vi "直通基准_数据库操作.vi"(8 "出口":i32, 9 "进口":i32, 11 "Freq&S":T1) -> ()   [LabVIEW 2015]
uses:
  network_Global/Global.vi
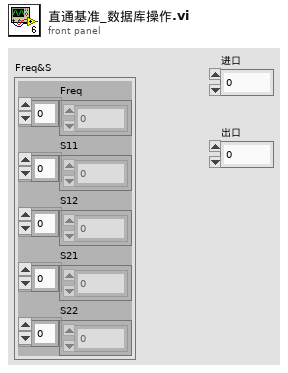
[diagram p1: front panel]
types:
  T1 = cluster{"Freq":dbl[], "S11":dbl[], "S12":dbl[], "S21":dbl[], "S22":dbl[]}
  T2 = typedef "测试类型.ctl" = u16
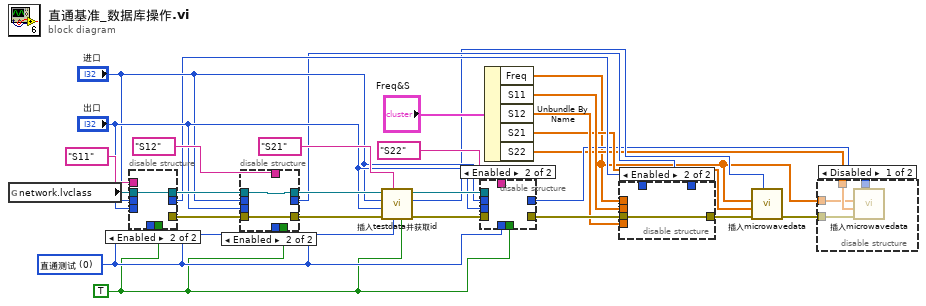
[diagram p0: block diagram]
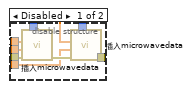
[diagram p3: hidden frame]
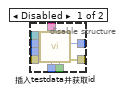
[diagram p4: hidden frame]
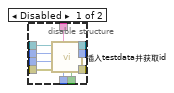
[diagram p5: hidden frame]
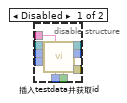
[diagram p6: hidden frame]
diagram:
  w2 = T2 0 items=["直通测试", "校准测试", "电缆"] ("测试类型")
  w1 = TRUE ("Ref")
  n1 = global read "Global.vi" "network.lvclass"() -> (w28:refnum<class "network.lvclass">)
  n2 = disable-structure shown="Enabled" {
    disable-tunnel: w28 -> [w37 w38]
    disable-tunnel: [w36 w38] -> w20
    disable-tunnel: [w35 _] -> w19
    disable-tunnel: "S11" ("Combo Box") -> [w34 _]
    disable-tunnel: "出口" -> [w33 _]
    disable-tunnel: "进口" -> [w32 _]
    disable-tunnel: [w31 _] -> w14
    disable-tunnel: w2 -> [w30 _]
    disable-tunnel: w1 -> [w29 _]
    frame Disabled {
      n3 = call "插入testdata并获取id.vi"("Ref"=w29, "测试类型"=w30, "数据类型"=w34, "出口"=w33, "进口"=w32, "network in"=w37) -> ("error out"=w35:errorcluster, "id"=w31:i32, "network out"=w36:refnum<class "network.lvclass">)  [unwired: 3 in]
    }
    frame Enabled {
    }
  }
  n4 = disable-structure shown="Enabled" {
    disable-tunnel: "S12" ("Combo Box") -> [w48 _]
    disable-tunnel: [w47 w50] -> w22
    disable-tunnel: [w46 w49] -> w21
    disable-tunnel: w20 -> [w45 w49]
    disable-tunnel: w19 -> [w44 w50]
    disable-tunnel: "出口" -> [w43 _]
    disable-tunnel: "进口" -> [w42 _]
    disable-tunnel: [w41 _] -> w10
    disable-tunnel: w2 -> [w40 _]
    disable-tunnel: w1 -> [w39 _]
    frame Disabled {
      n5 = call "插入testdata并获取id.vi"("Ref"=w39, "测试类型"=w40, "数据类型"=w48, "error in (no error)"=w44, "出口"=w43, "进口"=w42, "network in"=w45) -> ("error out"=w47:errorcluster, "id"=w41:i32, "network out"=w46:refnum<class "network.lvclass">)  [unwired: 2 in]
    }
    frame Enabled {
    }
  }
  n6 = call "插入testdata并获取id.vi"("Ref"=w1, "测试类型"=w2, "数据类型"="S21" ("Combo Box"), "error in (no error)"=w22, "出口"="出口", "进口"="进口", "network in"=w21) -> ("error out"=w24:errorcluster, "id"=w7:i32, "network out"=w23:refnum<class "network.lvclass">)  [unwired: 2 in]
  n7 = disable-structure shown="Enabled" {
    disable-tunnel: "S22" ("Combo Box") -> [w59 _]
    disable-tunnel: w24 -> [w58 _]
    disable-tunnel: w23 -> [w57 _]
    disable-tunnel: "出口" -> [w56 _]
    disable-tunnel: "进口" -> [w55 _]
    disable-tunnel: [w54 _] -> w15
    disable-tunnel: [w53 _] -> w6
    disable-tunnel: w2 -> [w52 _]
    disable-tunnel: w1 -> [w51 _]
    frame Disabled {
      n8 = call "插入testdata并获取id.vi"("Ref"=w51, "测试类型"=w52, "数据类型"=w59, "error in (no error)"=w58, "出口"=w56, "进口"=w55, "network in"=w57) -> ("error out"=w54:errorcluster, "id"=w53:i32)  [unwired: 2 in, 1 out]
    }
    frame Enabled {
    }
  }
  n9 = Unbundle By Name("Freq&S") -> ("Freq"=w3:dbl[], "S11"=w12:dbl[], "S12"=w11:dbl[], "S21"=w8:dbl[], "S22"=w4:dbl[])
  n10 = disable-structure shown="Enabled" {
    disable-tunnel: w15 -> [w67 w68]
    disable-tunnel: w14 -> [w66 _]
    disable-tunnel: w12 -> [w64 _]
    disable-tunnel: w11 -> [w63 _]
    disable-tunnel: w10 -> [w62 _]
    disable-tunnel: [w61 w68] -> w9
    disable-tunnel: w3 -> [w60 _]
    frame Disabled {
      n11 = call "插入microwavedata.vi"("pid"=w66, "error in"=w67, "S-Parameter"=w64, "freq"=w60) -> ("error out"=w65:errorcluster)  [unwired: 7 in]
      n12 = call "插入microwavedata.vi"("pid"=w62, "error in"=w65, "S-Parameter"=w63, "freq"=w60) -> ("error out"=w61:errorcluster)  [unwired: 7 in]
    }
    frame Enabled {
    }
  }
  n13 = call "插入microwavedata.vi"("pid"=w7, "error in"=w9, "S-Parameter"=w8, "freq"=w3) -> ("error out"=w5:errorcluster)  [unwired: 7 in]
  n14 = disable-structure shown="Disabled" {
    disable-tunnel: w6 -> [w72 _]
    disable-tunnel: w5 -> [w71 _]
    disable-tunnel: w4 -> [w70 _]
    disable-tunnel: w3 -> [w69 _]
    frame Disabled {
      n15 = call "插入microwavedata.vi"("pid"=w72, "error in"=w71, "S-Parameter"=w70, "freq"=w69) -> ()  [unwired: 7 in, 1 out]
    }
    frame Enabled {
    }
  }
